vi "Calibrate RT Parameters 2 Ticks (uSMC).vi"(2 "RTMinError (a.u.)":u16, 3 "RTDelta (a.u.)":u16) -> (0 "RTMinError (ticks)":u16, 1 "RTDelta (ticks)":u16)   [LabVIEW 2010, in "SignalWriterMH110203USBStepperMotor.lvclass"]
uses:
  SignalWriterMH110203USBStepperMotor.lvclass
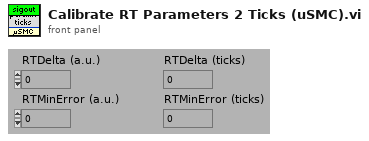
[diagram p1: front panel]
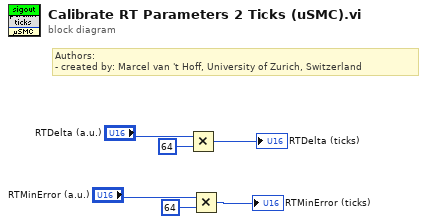
[diagram p0: block diagram]
diagram:
  # "Authors: \n- created by: Marcel van 't Hoff, University of Zurich, Switzerland"
  n1 = Multiply(x="RTDelta (a.u.)", y=u16 64) -> (x*y=→"RTDelta (ticks)":u16)
  n2 = Multiply(x="RTMinError (a.u.)", y=u16 64) -> (x*y=→"RTMinError (ticks)":u16)
